vi "探头模板-16-24.vi"() -> ()   [LabVIEW 2017]
panel:
  in  "停止":bool=TRUE
  out "探头地址":T1(ring)
  out "探头信息":string
  in  "显示限值？":bool=TRUE
  out "测量值":dbl format="%.2g"
  out "探头状态":T2(ring)=enum."离线"
  out "单位":enum16{"μSv/h", "mSv/h"}(ring)
  out "限值1":string="一级限值："
  out "限值2":string="二级限值："
  in  "数据簇":T3
  out "累积剂量":string="二级限值："
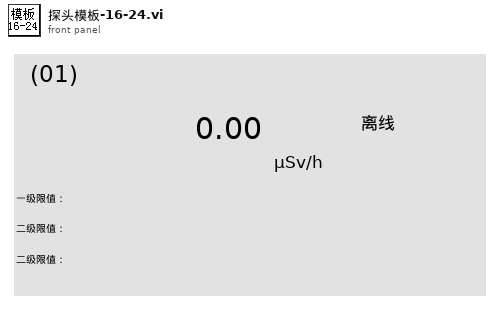
[diagram p1: front panel]
types:
  T1 = enum16{"(01)", "(02)", "(03)", "(04)", "(05)", "(06)", "(07)", "(08)", "(09)", "(10)", "(11)", "(12)", "(13)", "(14)", "(15)", "(16)", "(17)", "(18)", "(19)", "(20)", "(21)", "(22)", "(23)", "(24)", "(25)", "(26)", "(27)", "(28)", "(29)", "(30)", "(31)", "(32)", "(33)", "(34)", "(35)"}
  T2 = enum16{"正常", "未启用", "离线", "一级报警", "二级报警", "累积报警"}
  T3 = cluster{"启用状态？":bool, "测量值":cluster{"X":timestamp, "Y":dbl}, "限值簇":cluster{"限值1":dbl, "限值2":dbl, "探头限值":enum16{"一级限值", "二级限值"}}, "报警状态":enum16{"正常", "一级报警", "二级报警", "累积报警"}, "探头信息":string, "探头地址":i32, "累积剂量":cluster{"设备名称":string, "启用累积？":bool, "起始时间":timestamp, "累积剂量":dbl, "累积报警阈值":dbl}}
  T4 = cluster{"限值1":dbl, "限值2":dbl, "探头限值":enum16{"一级限值", "二级限值"}}
  T5 = cluster{"设备名称":string, "启用累积？":bool, "起始时间":timestamp, "累积剂量":dbl, "累积报警阈值":dbl}
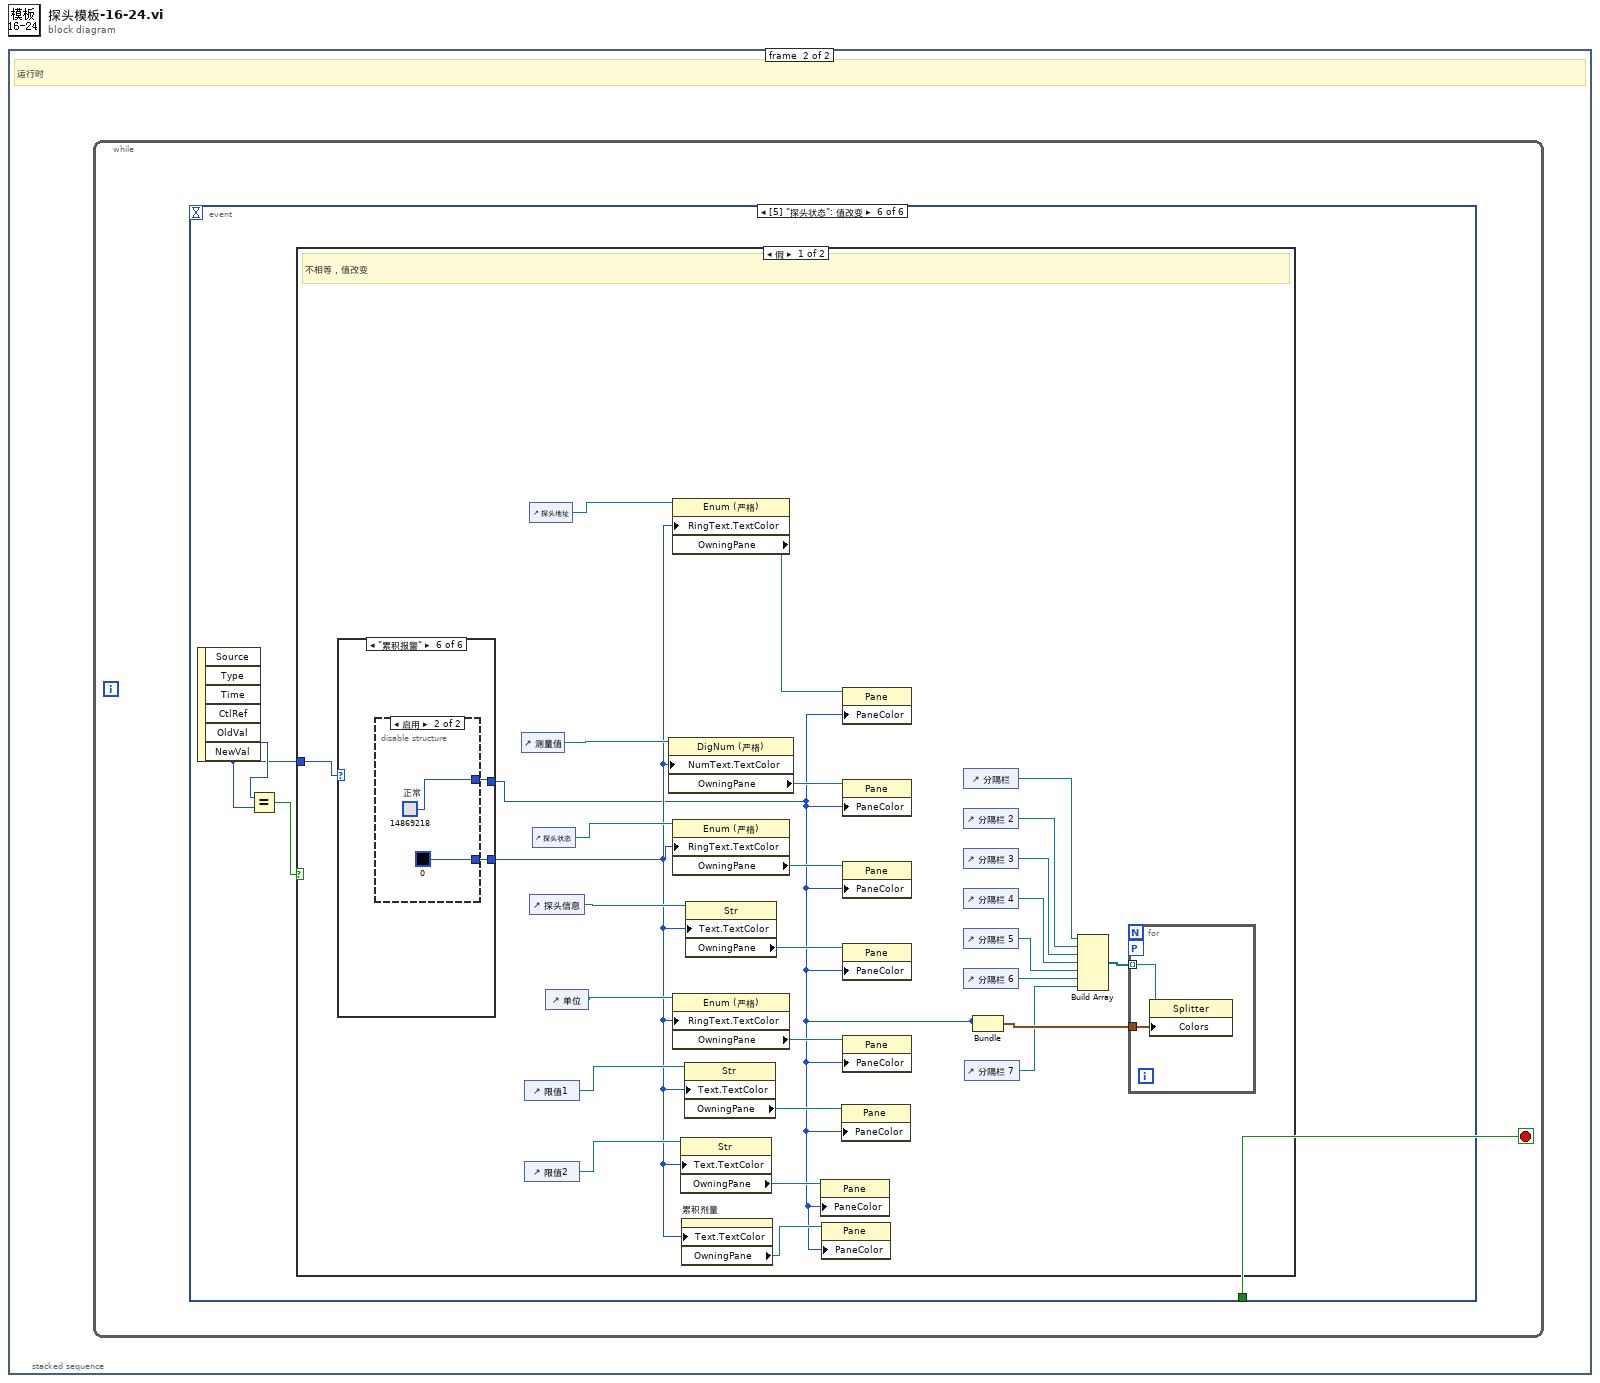
[diagram p0: block diagram]
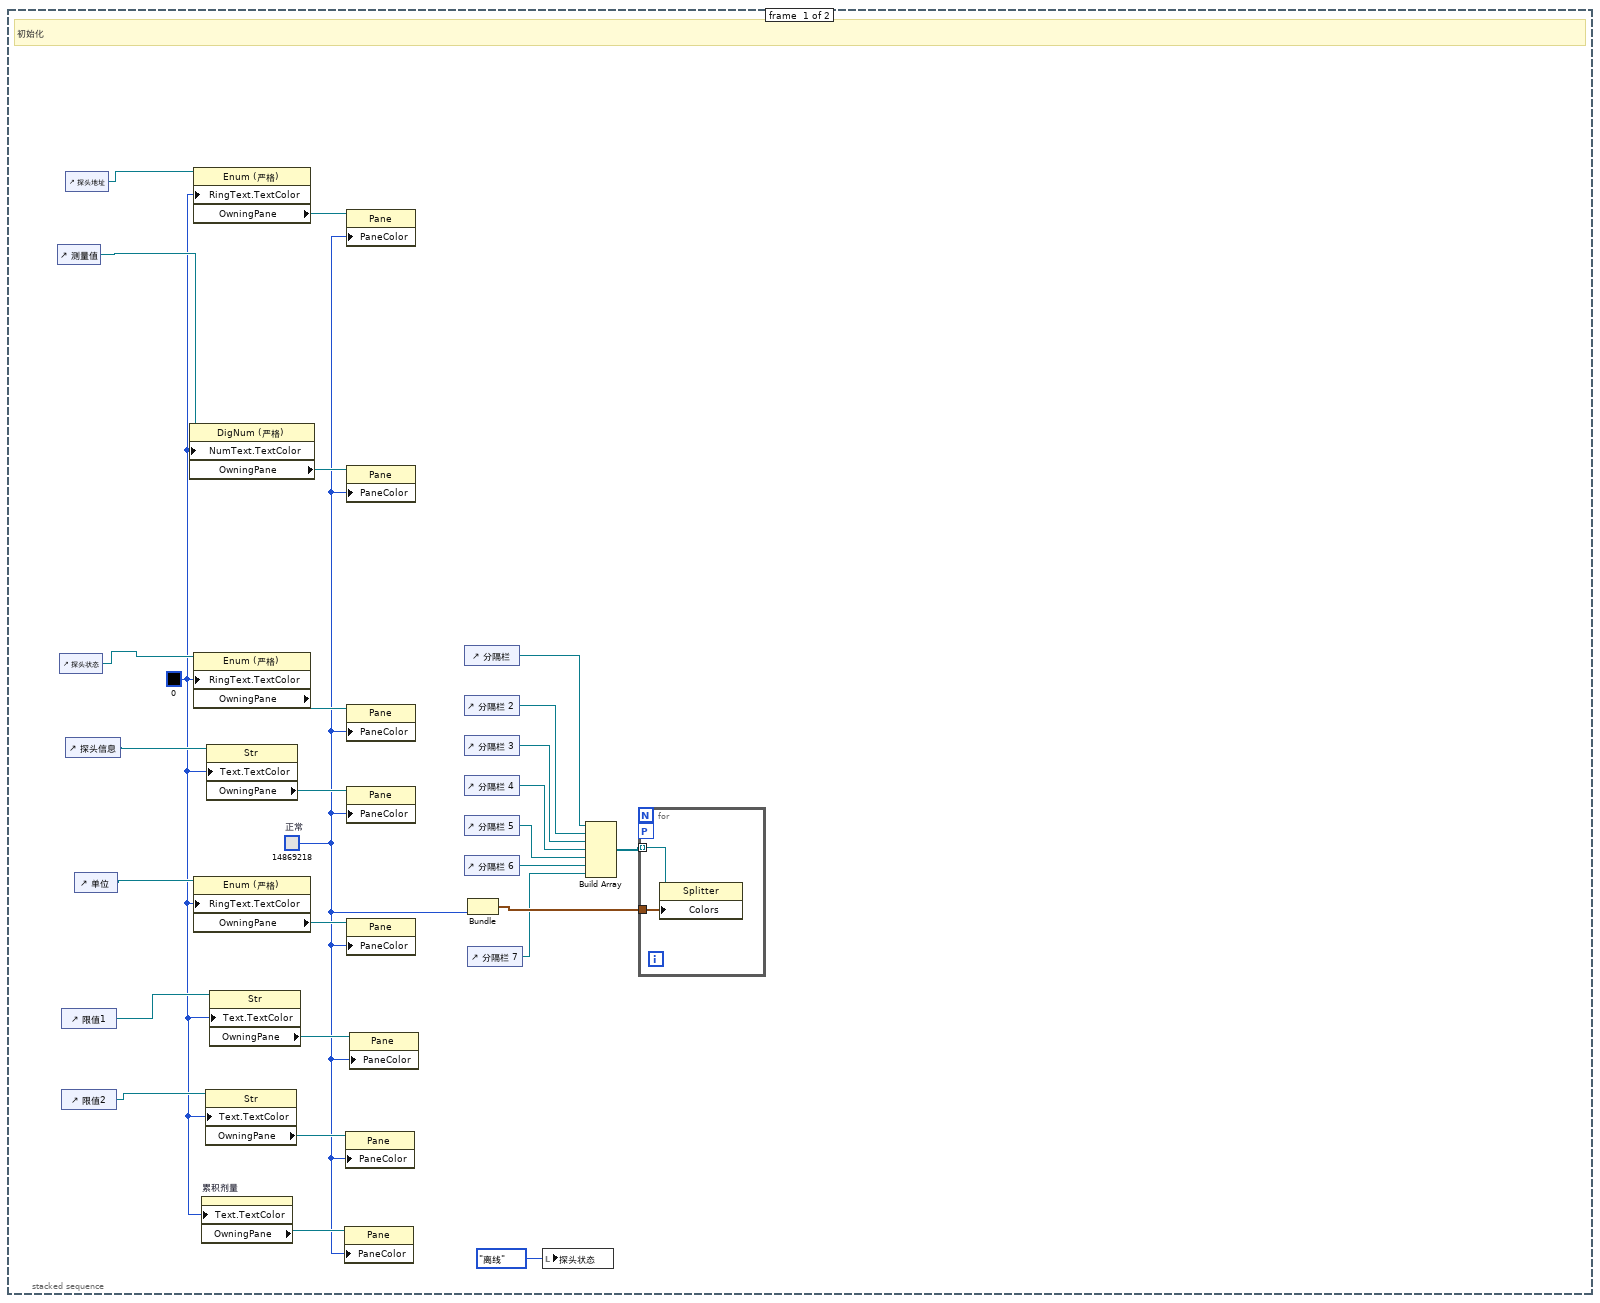
[diagram p2: hidden frame]
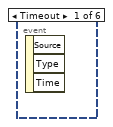
[diagram p3: hidden frame]
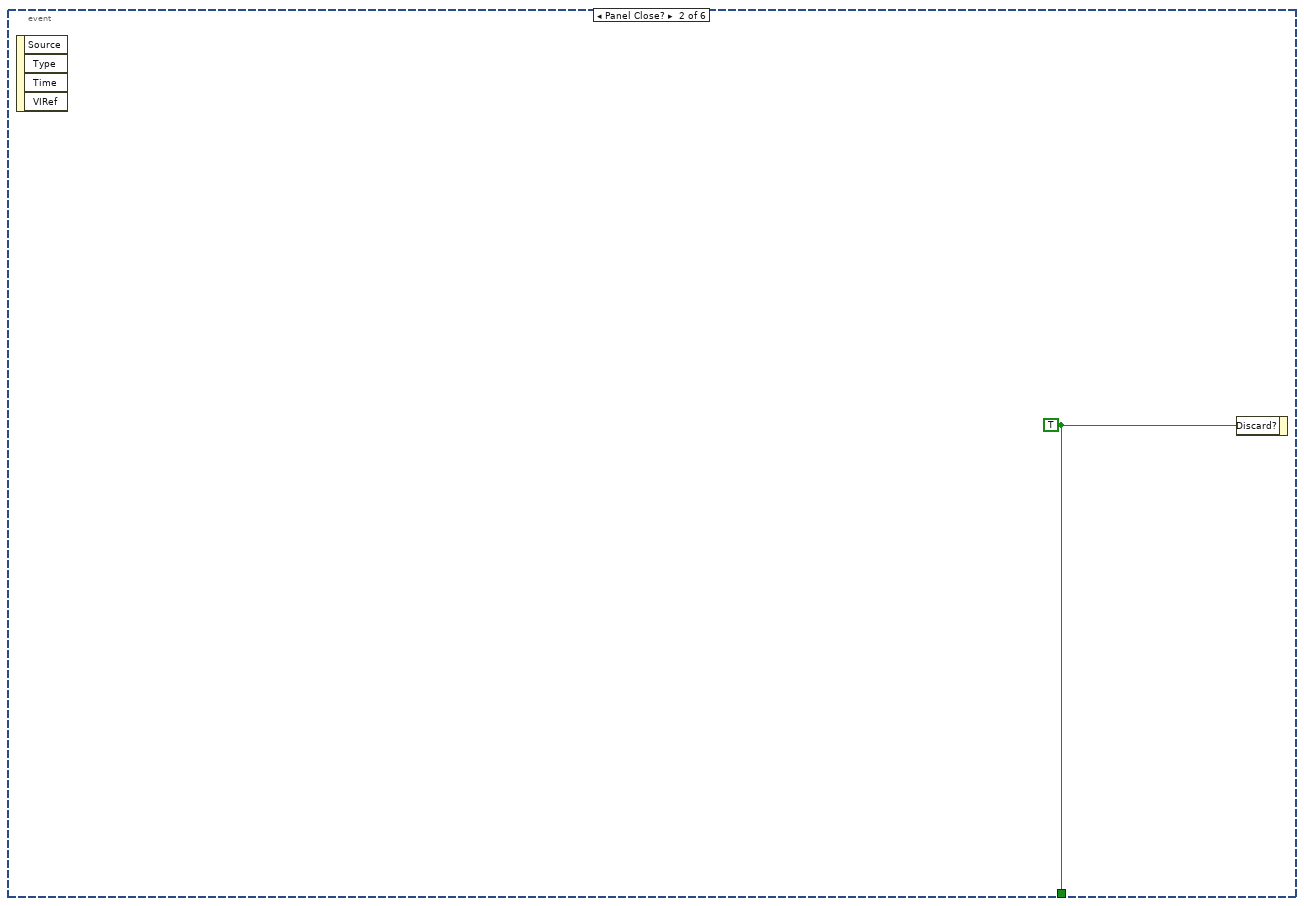
[diagram p4: hidden frame]
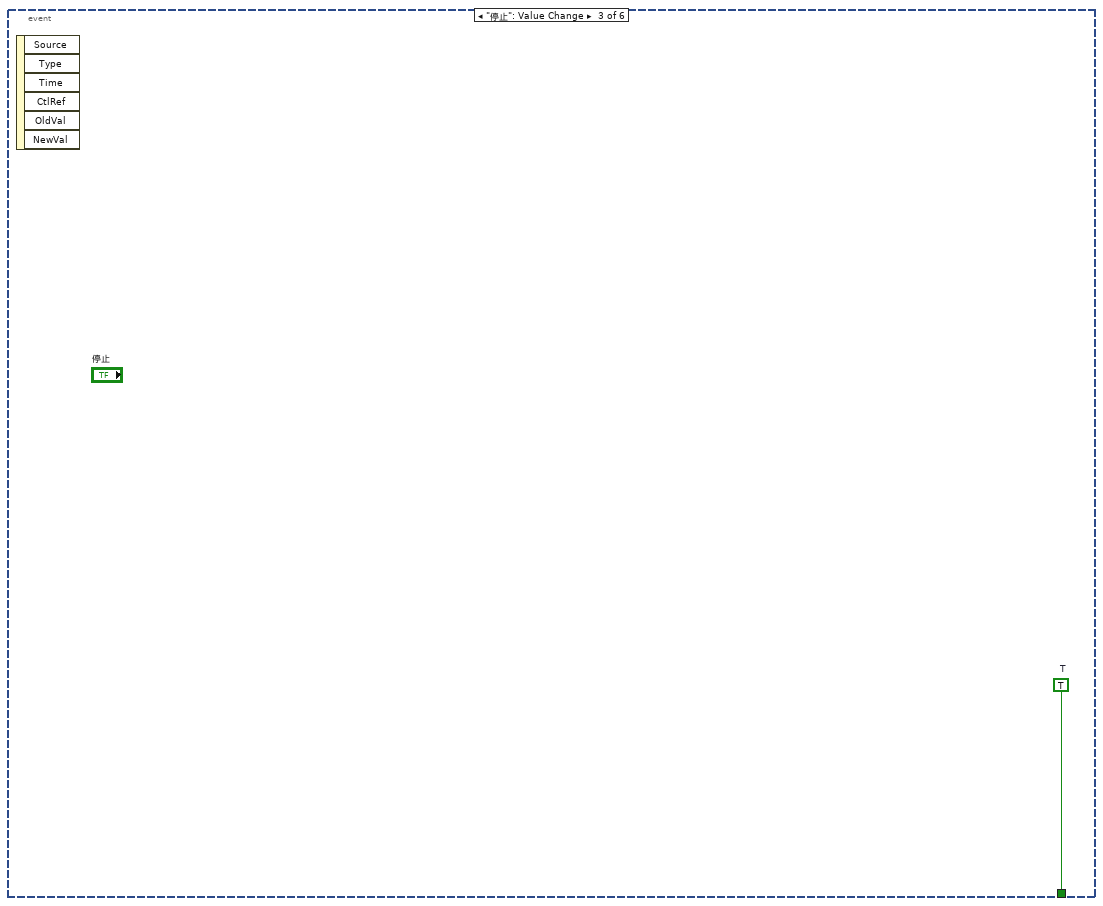
[diagram p5: hidden frame]
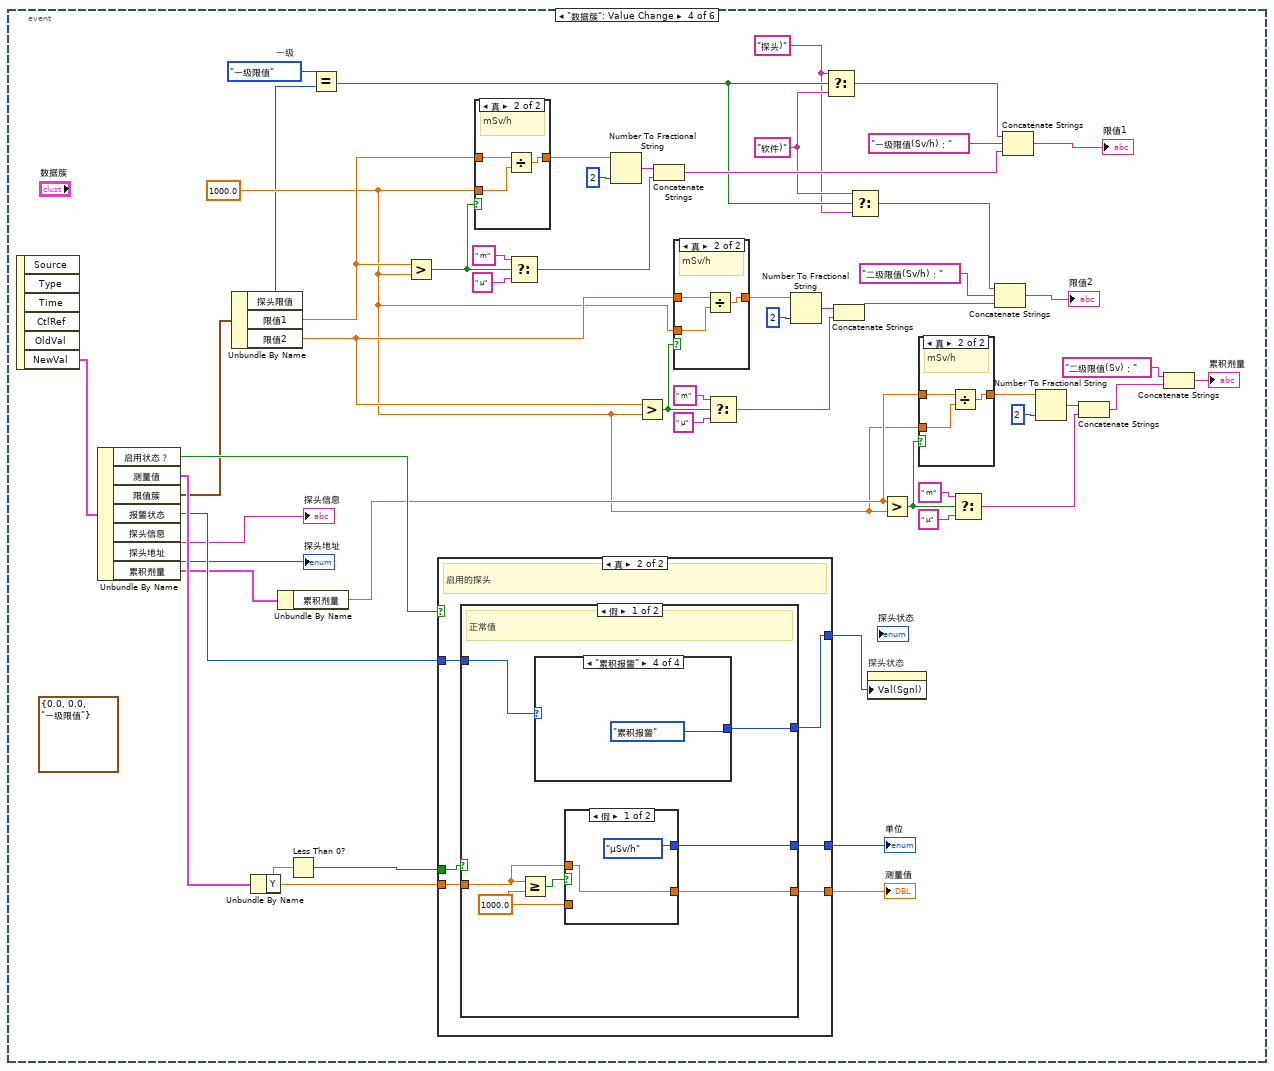
[diagram p6: hidden frame]
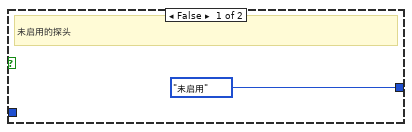
[diagram p10: hidden frame]
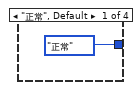
[diagram p11: hidden frame]
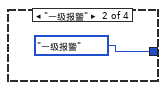
[diagram p12: hidden frame]
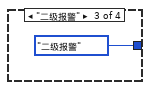
[diagram p13: hidden frame]
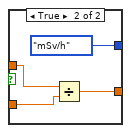
[diagram p14: hidden frame]
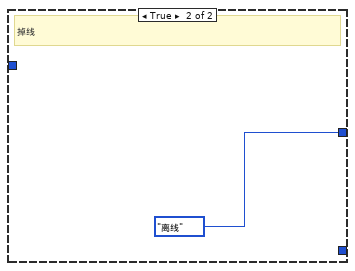
[diagram p15: hidden frame]
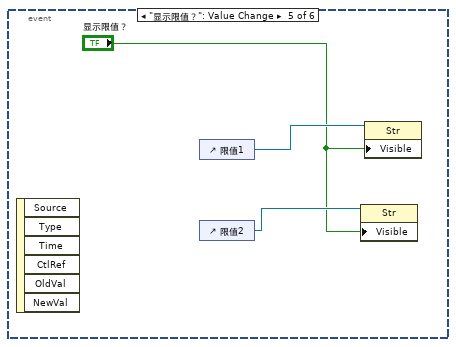
[diagram p16: hidden frame]
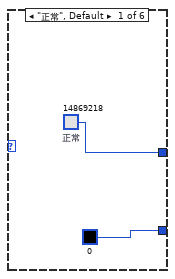
[diagram p17: hidden frame]
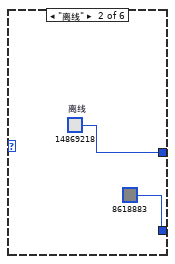
[diagram p18: hidden frame]
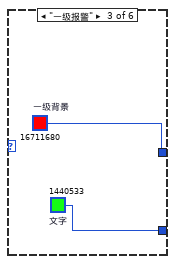
[diagram p19: hidden frame]
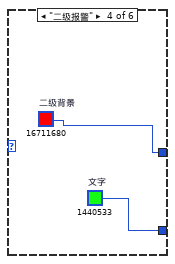
[diagram p20: hidden frame]
diagram:
  n1 = stacked-sequence {
    frame #0 {
      w1 = u32 0
      w3 = u32 14869218  # 正常
      # "初始化"
      n2 = control-ref of="测量值"() -> (w19:refnum<vi>)
      n3 = control-ref of="探头状态"() -> (w18:refnum<vi>)
      n4 = control-ref of="限值1"() -> (w12:refnum<vi>)
      n5 = control-ref of="限值2"() -> (w13:refnum<vi>)
      n6 = control-ref of="探头地址"() -> (w20:refnum<vi>)
      n7 = control-ref of="探头信息"() -> (w17:refnum<vi>)
      n8 = control-ref of="单位"() -> (w16:refnum<vi>)
      n9 = property on="属性节点" class="DigNum (严格)"(reference=w19, "NumText.TextColor"=w1) -> ("OwningPane"=w26:refnum<vi>)  [unwired: 1 in, 2 out]
      n10 = property on="属性节点" class="Enum (严格)"(reference=w20, "RingText.TextColor"=w1) -> ("OwningPane"=w27:refnum<vi>)  [unwired: 1 in, 2 out]
      n11 = property on="属性节点" class="Enum (严格)"(reference=w18, "RingText.TextColor"=w1) -> ("OwningPane"=w25:refnum<vi>)  [unwired: 1 in, 2 out]
      n12 = property on="属性节点" class="Enum (严格)"(reference=w16, "RingText.TextColor"=w1) -> ("OwningPane"=w23:refnum<vi>)  [unwired: 1 in, 2 out]
      n13 = property on="累积剂量" class="Str"("Text.TextColor"=w1) -> ("OwningPane"=w4:refnum<vi>)  [unwired: 2 in, 2 out]
      n14 = property on="属性节点" class="Str"(reference=w13, "Text.TextColor"=w1) -> ("OwningPane"=w14:refnum<vi>)  [unwired: 1 in, 2 out]
      n15 = property on="属性节点" class="Str"(reference=w17, "Text.TextColor"=w1) -> ("OwningPane"=w24:refnum<vi>)  [unwired: 1 in, 2 out]
      n16 = property on="属性节点" class="Str"(reference=w12, "Text.TextColor"=w1) -> ("OwningPane"=w15:refnum<vi>)  [unwired: 1 in, 2 out]
      n17 = property class="Pane"(reference=w4, "PaneColor"=w3) -> ()  [unwired: 1 in, 2 out]
      n18 = property class="Pane"(reference=w14, "PaneColor"=w3) -> ()  [unwired: 1 in, 2 out]
      n19 = property class="Pane"(reference=w27, "PaneColor"=w3) -> ()  [unwired: 1 in, 2 out]
      n20 = property class="Pane"(reference=w26, "PaneColor"=w3) -> ()  [unwired: 1 in, 2 out]
      n21 = property class="Pane"(reference=w25, "PaneColor"=w3) -> ()  [unwired: 1 in, 2 out]
      n22 = property class="Pane"(reference=w24, "PaneColor"=w3) -> ()  [unwired: 1 in, 2 out]
      n23 = property class="Pane"(reference=w23, "PaneColor"=w3) -> ()  [unwired: 1 in, 2 out]
      n24 = property class="Pane"(reference=w15, "PaneColor"=w3) -> ()  [unwired: 1 in, 2 out]
      n25 = control-ref of="分隔栏"() -> (w11:refnum<vi>)
      n26 = control-ref of="分隔栏 2"() -> (w10:refnum<vi>)
      n27 = control-ref of="分隔栏 3"() -> (w9:refnum<vi>)
      n28 = control-ref of="分隔栏 4"() -> (w8:refnum<vi>)
      n29 = control-ref of="分隔栏 5"() -> (w7:refnum<vi>)
      n30 = control-ref of="分隔栏 6"() -> (w6:refnum<vi>)
      n31 = Bundle("正常"=w3, "正常"=w3) -> (w22:cluster{"正常":u32, "正常":u32})  [unwired: 1 in]
      n32 = control-ref of="分隔栏 7"() -> (w2:refnum<vi>)
      n33 = local write "探头状态"(enum16{"正常", "未启用", "离线", "一级报警", "二级报警"}."离线" ("探头状态")) -> ()
      n34 = Build Array(w11, w10, w9, w8, w7, w6, w2) -> (w5:refnum<vi>[])
      n35 = for {
        tunnel: w22 -> [w29]
        workers-P: _ -> [_]
        tunnel: w5 -> [w28] mode=indexing
        n36 = property on="属性节点" class="Splitter"(reference=w28, "Colors"=w29) -> ()  [unwired: 1 in, 2 out]
      }
    }
    frame #1 {
      # "运行时"
      n37 = while {
        stop <- w30 stop-if-true
        n38 = event shown="[5] \"探头状态\": 值改变" {
          selector: _ -> [_ _ _ _ _ _]
          dyn-events: _ -> [_ _ _ _ _ _]
          timeout: _ -> [_ _ _ _ _ _]
          tunnel: [_ w31 w32 _ _ _] -> w30
          event Timeout {
            n39 = event-data() -> ()  [unwired: 1 in, 3 out]
          }
          event Panel Close? {
            w31 = TRUE ("放弃？")
            n40 = event-data() -> ()  [unwired: 1 in, 4 out]
            n41 = event-data("Discard?"=w31) -> ()  [unwired: 1 in, 1 out]
          }
          event "停止": Value Change {
            w32 = TRUE  # T
            n42 = event-data() -> ()  [unwired: 1 in, 6 out]
          }
          event "数据簇": Value Change {
            w36 = "软件)" ("字符串")
            w35 = "探头)" ("字符串")
            w38 = enum16{"一级限值", "二级限值"}."一级限值"  # 一级
            (unwired) T4 {"限值1"=0.0, "限值2"=0.0, "探头限值"=enum."一级限值"} ("探头限值簇")
            w41 = 1000.0 ("y")
            n43 = event-data() -> ("NewVal"=w86:T3)  [unwired: 1 in, 5 out]
            n44 = Unbundle By Name(w86) -> ("启用状态？"=w82:bool, "测量值"=w83:cluster{"X":timestamp, "Y":dbl}, "限值簇"=w55:T4, "报警状态"=w81:enum16{"正常", "一级报警", "二级报警", "累积报警"}, "探头信息"=→"探头信息":string, "探头地址"=→"探头地址":i32, "累积剂量"=w43:T5)
            n45 = Unbundle By Name(w55) -> ("探头限值"=w39:enum16{"一级限值", "二级限值"}, "限值1"=w72:dbl, "限值2"=w74:dbl)
            n46 = Unbundle By Name(w83) -> ("Y"=w85:dbl)
            n47 = Unbundle By Name(w43) -> ("累积剂量"=w42:dbl)
            n48 = Less Than 0?(x=w85) -> (x < 0?=w84:bool)
            n49 = Equal?(x=w38, y=w39) -> (x = y?=w37:bool)
            n50 = Greater?(x=w72, y=w41) -> (0:w59:bool)
            n51 = case shown="真" w82 {
              tunnel: w84 -> [_ w105]
              tunnel: w85 -> [_ w104]
              tunnel: [_ w103] -> w78
              tunnel: [_ w102] -> w77
              tunnel: [enum16{"正常", "未启用", "离线", "一级报警", "二级报警"}."未启用" ("探头状态") w101] -> w76
              tunnel: w81 -> [_ w100]
              frame False {
                # "未启用的探头"
              }
              frame True {
                # "启用的探头"
                n52 = case shown="假" w105 {
                  tunnel: w104 -> [w111 _]
                  tunnel: [w109 _] -> w103
                  tunnel: [w108 _] -> w102
                  tunnel: [w106 enum16{"正常", "未启用", "离线", "一级报警", "二级报警"}."离线" ("探头状态")] -> w101
                  tunnel: w100 -> [w107 _]
                  frame False {
                    w110 = 1000.0 ("y")
                    # "正常值"
                    n53 = Greater Or Equal?(x=w111, y=w110) -> (x >= y?=w112:bool)
                    n54 = case shown="\"累积报警\"" w107 {
                      tunnel: [enum16{"正常", "未启用", "离线", "一级报警", "二级报警"}."正常" ("探头状态") enum16{"正常", "未启用", "离线", "一级报警", "二级报警"}."一级报警" ("探头状态") enum16{"正常", "未启用", "离线", "一级报警", "二级报警"}."二级报警" ("探头状态") T2."累积报警" ("探头状态")] -> w106
                      frame "正常", Default {
                      }
                      frame "一级报警" {
                      }
                      frame "二级报警" {
                      }
                      frame "累积报警" {
                      }
                    }
                    n55 = case shown="假" w112 {
                      tunnel: w111 -> [w118 w122]
                      tunnel: w110 -> [_ w121]
                      tunnel: [w118 w120] -> w109
                      tunnel: [enum16{"μSv/h", "mSv/h"}."μSv/h" ("单位") enum16{"μSv/h", "mSv/h"}."mSv/h" ("单位")] -> w108
                      frame False {
                      }
                      frame True {
                        n56 = Divide(x=w122, y=w121) -> (x/y=w120:dbl)
                      }
                    }
                  }
                  frame True {
                    # "掉线"
                  }
                }
              }
            }
            "测量值" <- w78
            "单位" <- w77
            n57 = case shown="真" w59 {
              tunnel: w72 -> [w95 w98]
              tunnel: w41 -> [_ w97]
              tunnel: [w95 w96] -> w64
              frame False {
                # "uSv/h"
              }
              frame True {
                # "mSv/h"
                n58 = Divide(x=w98, y=w97) -> (x/y=w96:dbl)
              }
            }
            n59 = Select(t=" m" ("F-格式字符串"), s=w59, f=" μ" ("F-格式字符串")) -> (s? t:f=w63:string)
            n60 = Number To Fractional String(number=w64, precision (6)=i16 2 ("精度(6)")) -> (F-format string=w60:string)  [unwired: 2 in]
            n61 = Greater?(x=w74, y=w41) -> (0:w66:bool)
            n62 = Concatenate Strings(w60, w63) -> (w73:string)
            n63 = case shown="真" w66 {
              tunnel: w74 -> [w91 w94]
              tunnel: w41 -> [_ w93]
              tunnel: [w91 w92] -> w71
              frame False {
                # "uSv/h"
              }
              frame True {
                # "mSv/h"
                n64 = Divide(x=w94, y=w93) -> (x/y=w92:dbl)
              }
            }
            n65 = Select(t=" m" ("F-格式字符串"), s=w66, f=" μ" ("F-格式字符串")) -> (s? t:f=w70:string)
            n66 = Number To Fractional String(number=w71, precision (6)=i16 2 ("精度(6)")) -> (F-format string=w67:string)  [unwired: 2 in]
            n67 = Select(t=w35, s=w37, f=w36) -> (s? t:f=w34:string)
            n68 = Concatenate Strings(w67, w70) -> (w75:string)
            n69 = Select(t=w36, s=w37, f=w35) -> (s? t:f=w33:string)
            n70 = property on="探头状态" class="Enum (严格)"("Val(Sgnl)"=w76) -> ()  [unwired: 2 in, 2 out]
            n71 = Greater?(x=w42, y=w41) -> (0:w51:bool)
            n72 = case shown="真" w51 {
              tunnel: w42 -> [w87 w90]
              tunnel: w41 -> [_ w89]
              tunnel: [w87 w88] -> w46
              frame False {
                # "uSv/h"
              }
              frame True {
                # "mSv/h"
                n73 = Divide(x=w90, y=w89) -> (x/y=w88:dbl)
              }
            }
            n74 = Select(t=" m" ("F-格式字符串"), s=w51, f=" μ" ("F-格式字符串")) -> (s? t:f=w47:string)
            n75 = Concatenate Strings(w33, "二级限值(Sv/h)：" ("字符串"), w75) -> (→"限值2":string)
            n76 = Concatenate Strings(w34, "一级限值(Sv/h)：" ("字符串"), w73) -> (→"限值1":string)
            n77 = Number To Fractional String(number=w46, precision (6)=i16 2 ("精度(6)")) -> (F-format string=w50:string)  [unwired: 2 in]
            n78 = Concatenate Strings(w50, w47) -> (w44:string)
            n79 = Concatenate Strings("二级限值(Sv)：" ("字符串"), w44) -> (→"累积剂量":string)
          }
          event "显示限值？": Value Change {
            n80 = event-data() -> ()  [unwired: 1 in, 6 out]
            n81 = control-ref of="限值1"() -> (w125:refnum<vi>)
            n82 = control-ref of="限值2"() -> (w126:refnum<vi>)
            n83 = property on="属性节点" class="Str"(reference=w126, "Visible"="显示限值？") -> ()  [unwired: 1 in, 2 out]
            n84 = property on="属性节点" class="Str"(reference=w125, "Visible"="显示限值？") -> ()  [unwired: 1 in, 2 out]
          }
          event "探头状态": Value Change {
            n85 = event-data() -> ("OldVal"=w129:T2, "NewVal"=w127:T2)  [unwired: 1 in, 4 out]
            n86 = Equal?(x=w129, y=w127) -> (x = y?=w128:bool)
            n87 = case shown="假" w128 {
              tunnel: w127 -> [w143 _]
              frame False {
                # "不相等，值改变"
                n88 = case shown="\"累积报警\"" w143 {
                  tunnel: [w157 w159 w162 w164 w165 w168] -> w131
                  tunnel: [u32 0 u32 8618883 w161 w163 w166 w167] -> w132
                  frame "正常", Default {
                    w157 = u32 14869218  # 正常
                  }
                  frame "离线" {
                    w159 = u32 14869218  # 离线
                  }
                  frame "一级报警" {
                    w161 = u32 1440533  # 文字
                    w162 = u32 16711680  # 一级背景
                  }
                  frame "二级报警" {
                    w163 = u32 1440533  # 文字
                    w164 = u32 16711680  # 二级背景
                  }
                  frame "未启用" {
                    w165 = u32 14869218  # 正常
                    w166 = u32 6579300  # 禁用
                  }
                  frame "累积报警" {
                    n89 = disable-structure shown="启用" {
                      disable-tunnel: [w170 w172] -> w168
                      disable-tunnel: [w169 u32 0] -> w167
                      frame Disabled {
                        w169 = u32 1440533  # 文字
                        w170 = u32 16711680  # 一级背景
                      }
                      frame Enabled {
                        w172 = u32 14869218  # 正常
                      }
                    }
                  }
                }
                n90 = control-ref of="测量值"() -> (w147:refnum<vi>)
                n91 = control-ref of="限值1"() -> (w135:refnum<vi>)
                n92 = control-ref of="限值2"() -> (w134:refnum<vi>)
                n93 = control-ref of="探头地址"() -> (w148:refnum<vi>)
                n94 = control-ref of="探头信息"() -> (w145:refnum<vi>)
                n95 = control-ref of="探头状态"() -> (w146:refnum<vi>)
                n96 = control-ref of="单位"() -> (w144:refnum<vi>)
                n97 = property on="属性节点" class="DigNum (严格)"(reference=w147, "NumText.TextColor"=w132) -> ("OwningPane"=w155:refnum<vi>)  [unwired: 1 in, 2 out]
                n98 = property on="属性节点" class="Enum (严格)"(reference=w148, "RingText.TextColor"=w132) -> ("OwningPane"=w156:refnum<vi>)  [unwired: 1 in, 2 out]
                n99 = property on="属性节点" class="Enum (严格)"(reference=w146, "RingText.TextColor"=w132) -> ("OwningPane"=w154:refnum<vi>)  [unwired: 1 in, 2 out]
                n100 = property on="属性节点" class="Enum (严格)"(reference=w144, "RingText.TextColor"=w132) -> ("OwningPane"=w152:refnum<vi>)  [unwired: 1 in, 2 out]
                n101 = property on="属性节点" class="Str"(reference=w134, "Text.TextColor"=w132) -> ("OwningPane"=w136:refnum<vi>)  [unwired: 1 in, 2 out]
                n102 = property on="累积剂量" class="Str"("Text.TextColor"=w132) -> ("OwningPane"=w133:refnum<vi>)  [unwired: 2 in, 2 out]
                n103 = property on="属性节点" class="Str"(reference=w135, "Text.TextColor"=w132) -> ("OwningPane"=w137:refnum<vi>)  [unwired: 1 in, 2 out]
                n104 = property on="属性节点" class="Str"(reference=w145, "Text.TextColor"=w132) -> ("OwningPane"=w153:refnum<vi>)  [unwired: 1 in, 2 out]
                n105 = property class="Pane"(reference=w136, "PaneColor"=w131) -> ()  [unwired: 1 in, 2 out]
                n106 = property class="Pane"(reference=w133, "PaneColor"=w131) -> ()  [unwired: 1 in, 2 out]
                n107 = property class="Pane"(reference=w137, "PaneColor"=w131) -> ()  [unwired: 1 in, 2 out]
                n108 = property class="Pane"(reference=w156, "PaneColor"=w131) -> ()  [unwired: 1 in, 2 out]
                n109 = property class="Pane"(reference=w155, "PaneColor"=w131) -> ()  [unwired: 1 in, 2 out]
                n110 = property class="Pane"(reference=w154, "PaneColor"=w131) -> ()  [unwired: 1 in, 2 out]
                n111 = property class="Pane"(reference=w153, "PaneColor"=w131) -> ()  [unwired: 1 in, 2 out]
                n112 = property class="Pane"(reference=w152, "PaneColor"=w131) -> ()  [unwired: 1 in, 2 out]
                n113 = control-ref of="分隔栏"() -> (w149:refnum<vi>)
                n114 = control-ref of="分隔栏 2"() -> (w142:refnum<vi>)
                n115 = control-ref of="分隔栏 3"() -> (w141:refnum<vi>)
                n116 = control-ref of="分隔栏 4"() -> (w140:refnum<vi>)
                n117 = control-ref of="分隔栏 5"() -> (w139:refnum<vi>)
                n118 = control-ref of="分隔栏 6"() -> (w138:refnum<vi>)
                n119 = control-ref of="分隔栏 7"() -> (w130:refnum<vi>)
                n120 = Bundle("正常"=w131, "正常"=w131) -> (w150:cluster{"正常":u32, "正常":u32})  [unwired: 1 in]
                n121 = Build Array(w149, w142, w141, w140, w139, w138, w130) -> (w151:refnum<vi>[])
                n122 = for {
                  tunnel: w150 -> [w174]
                  workers-P: _ -> [_]
                  tunnel: w151 -> [w173] mode=indexing
                  n123 = property on="属性节点" class="Splitter"(reference=w173, "Colors"=w174) -> ()  [unwired: 1 in, 2 out]
                }
              }
              frame True {
              }
            }
          }
        }
      }
    }
  }
